vi "get_allComponents.vi"(0 "HGF_Component in":refnum<class "HGF_Component.lvclass">, 5 "error in (no error)":errorcluster) -> (14 "HGF_Component out":refnum<class "HGF_Component.lvclass">, 16 "Components":refnum<class "HGF_Component.lvclass">[](array[class]), 19 "error out":errorcluster)   [LabVIEW 2014, in "HGF_BaseClasses.lvlib" / "HGF_Component.lvclass"]
doc: "Get a copy of all Components of Composite object of all hierarchy levels.\n\n<B>Attention:</B> This is a recursive dynamic dispatch VI."
uses:
  HGF_Component.lvclass
  HGF_Composite/HGF_Composite.lvclass
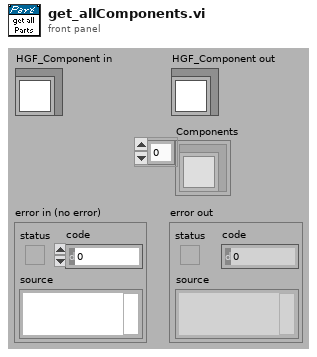
[diagram p1: front panel]
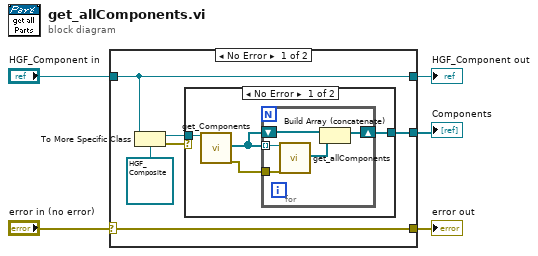
[diagram p0: block diagram]
diagram:
  n1 = case shown="No Error" "error in (no error)" {
    selector: "error in (no error)" -> [w11 w22]
    tunnel: [w11 w22] -> w4
    tunnel: [w10 w21] -> w2
    tunnel: "HGF_Component in" -> [w10 w21]
    tunnel: [w7 _] -> w1
    frame No Error {
      n2 = To More Specific Class(target class=refnum<class "HGF_Composite.lvclass"> refnum ("HGF_Composite.lvclass"), reference=w10) -> (specific class reference=w8:refnum<class "HGF_Composite.lvclass">, error out=w6:errorcluster)  [unwired: 1 in]
      n3 = case shown="No Error" w6 {
        tunnel: w8 -> [w15 _]
        tunnel: [w12 _] -> w7
        frame No Error {
          n4 = call "get_Components.vi"("HGF_Composite"=w15) -> ("Components"=w13:refnum<class "HGF_Component.lvclass">[], "error out"=w14:errorcluster)  [unwired: 1 in, 16 out]
          n5 = for {
            tunnel: w13 -> [w20] mode=indexing
            tunnel: w14 -> [w19]
            shift-right: [w17] -> w12
            shift-left: w13 -> [w18]
            n6 = call-dynamic "get_allComponents.vi"("HGF_Component in"=w20, "error in (no error)"=w19) -> ("Components"=w16:refnum<class "HGF_Component.lvclass">[])  [unwired: 17 out]
            n7 = Build Array (concatenate)(w18, w16) -> (w17:refnum<class "HGF_Component.lvclass">[])
          }
        }
        frame Error {
        }
      }
    }
    frame Error {
    }
  }
  "error out" <- w4
  "HGF_Component out" <- w2
  "Components" <- w1
